vi "new control rack tester.vi"() -> ()   [LabVIEW 2011]
uses:
  <vilib>/Utility/file.llb/Write To Spreadsheet File (DBL).vi
panel:
  out "ai0 8":dynamicdata(graph) caption="Helix Limited Current Set Point"
  in  "stop":bool
  out "ai0 16":dynamicdata(graph) caption="Torroidal Current Feedback"
  out "ai0 15":dynamicdata(graph) caption="Torroidal U Limit Set Point Buffered"
  out "ai0 14":dynamicdata(graph) caption="Torroidal Voltage Feedback"
  out "ai0 13":dynamicdata(graph) caption="Torroidal Voltage Feedback"
  out "ai0 12":dynamicdata(graph) caption="ECRH Reflection"
  out "ai0 11":dynamicdata(graph) caption="ECRH Power"
  out "ai0 10":dynamicdata(graph) caption="Torroidal U Limit Set Point"
  out "ai0 9":dynamicdata(graph) caption="Torroidal Limited Current Set Point"
  out "ai0 7":dynamicdata(graph) caption="Halpha Reserve Vin/10"
  out "ai0 6":dynamicdata(graph) caption="Torroidal Limited Current Set Point"
  out "ai0 5":dynamicdata(graph) caption="Helix Limited Current Set Point"
  out "ai0 4":dynamicdata(graph) caption="Helix Voltage Feedback"
  out "ai0 3":dynamicdata(graph) caption="Helix Current Feedback"
  out "ai0 2":dynamicdata(graph) caption="Helix U Limit Set Point Buffered"
  out "ai0":dynamicdata(graph) caption="Helix U Limit Set Point"
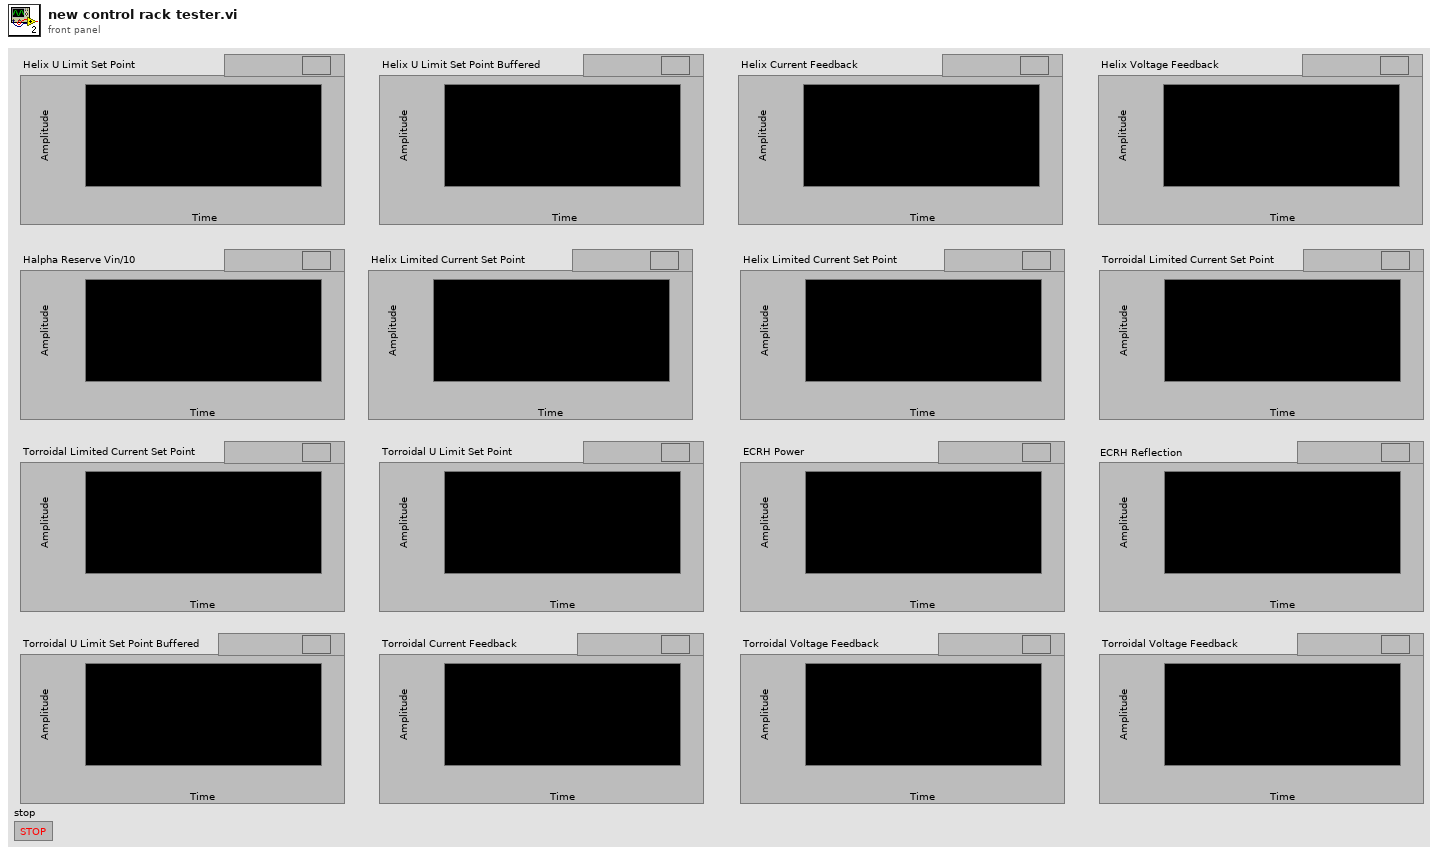
[diagram p1: front panel]
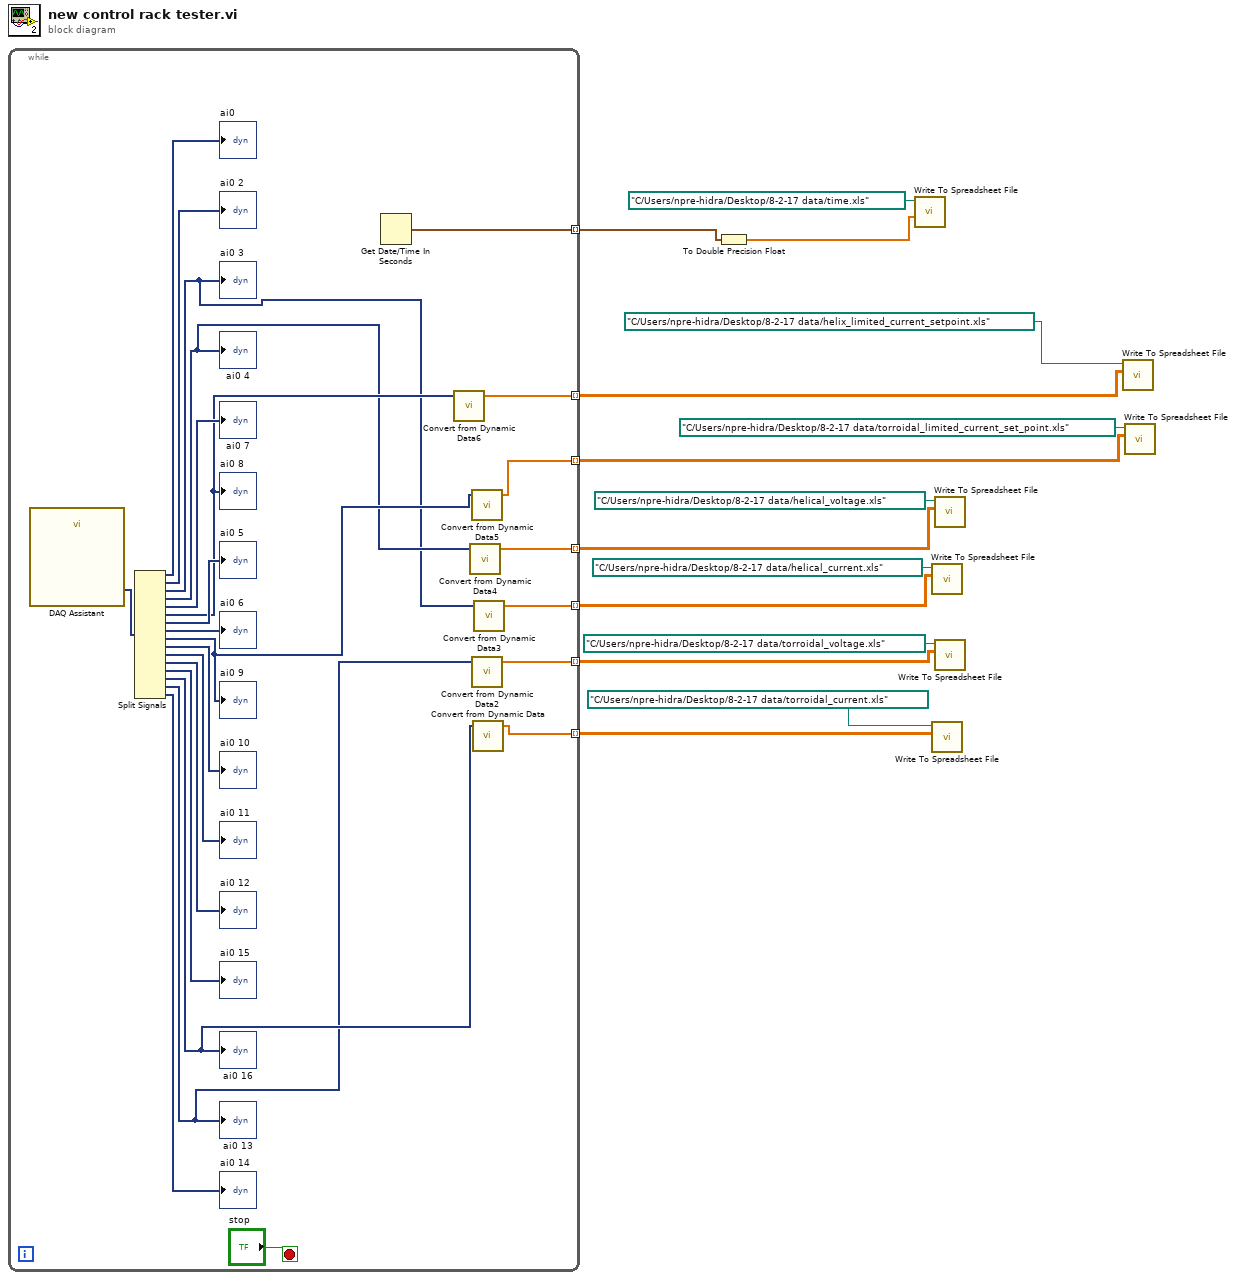
[diagram p0: block diagram]
diagram:
  n1 = while {
    tunnel: [w29] -> w14 mode=indexing
    tunnel: [w27] -> w8 mode=indexing
    tunnel: [w25] -> w6 mode=indexing
    tunnel: [w24] -> w5 mode=indexing
    tunnel: [w23] -> w4 mode=indexing
    tunnel: [w22] -> w3 mode=indexing
    tunnel: [w21] -> w2 mode=indexing
    stop <- "stop" stop-if-true
    n2 = call "DAQ Assistant"() -> ("data"=w30:dynamicdata)  [unwired: 17 in, 2 out]
    n3 = Split Signals(w30) -> (→"ai0":dynamicdata, →"ai0 2":dynamicdata, w17:dynamicdata, w18:dynamicdata, →"ai0 7":dynamicdata, w20:dynamicdata, →"ai0 5":dynamicdata, →"ai0 6":dynamicdata, w19:dynamicdata, →"ai0 10":dynamicdata, →"ai0 11":dynamicdata, →"ai0 12":dynamicdata, →"ai0 15":dynamicdata, w26:dynamicdata, w16:dynamicdata, →"ai0 14":dynamicdata)  [unwired: 16 in]
    "ai0 3" <- w17
    "ai0 4" <- w18
    "ai0 9" <- w19
    "ai0 13" <- w16
    "ai0 16" <- w26
    "ai0 8" <- w20
    n4 = Get Date/Time In Seconds() -> (seconds since 1Jan1904=w29:timestamp)
    n5 = call "Convert from Dynamic Data6"("Dynamic Data Type"=w20) -> ("Array"=w25:dbl[])  [unwired: 3 in]
    n6 = call "Convert from Dynamic Data4"("Dynamic Data Type"=w18) -> ("Array"=w23:dbl[])  [unwired: 3 in]
    n7 = call "Convert from Dynamic Data5"("Dynamic Data Type"=w19) -> ("Array"=w24:dbl[])  [unwired: 3 in]
    n8 = call "Convert from Dynamic Data2"("Dynamic Data Type"=w16) -> ("Array"=w21:dbl[])  [unwired: 3 in]
    n9 = call "Convert from Dynamic Data"("Dynamic Data Type"=w26) -> ("Array"=w27:dbl[])  [unwired: 3 in]
    n10 = call "Convert from Dynamic Data3"("Dynamic Data Type"=w17) -> ("Array"=w22:dbl[])  [unwired: 3 in]
  }
  n11 = To Double Precision Float(number=w14) -> (double precision float=w13:dbl[])
  n12 = call-poly <vilib>:"Write To Spreadsheet File.vi"("1D data"=w13, "file path (dialog if empty)"=path "C:/Users/npre-hidra/Desktop/8-2-17 data/time.xls") -> ()  [unwired: 6 in, 1 out]
  n13 = call-poly <vilib>:"Write To Spreadsheet File.vi"("2D data"=w3, "file path (dialog if empty)"=path "C:/Users/npre-hidra/Desktop/8-2-17 data/helical_current.xls") -> ()  [unwired: 6 in, 1 out]
  n14 = call-poly <vilib>:"Write To Spreadsheet File.vi"("2D data"=w8, "file path (dialog if empty)"=path "C:/Users/npre-hidra/Desktop/8-2-17 data/torroidal_current.xls") -> ()  [unwired: 6 in, 1 out]
  n15 = call-poly <vilib>:"Write To Spreadsheet File.vi"("2D data"=w4, "file path (dialog if empty)"=path "C:/Users/npre-hidra/Desktop/8-2-17 data/helical_voltage.xls") -> ()  [unwired: 6 in, 1 out]
  n16 = call-poly <vilib>:"Write To Spreadsheet File.vi"("2D data"=w2, "file path (dialog if empty)"=path "C:/Users/npre-hidra/Desktop/8-2-17 data/torroidal_voltage.xls") -> ()  [unwired: 6 in, 1 out]
  n17 = call-poly <vilib>:"Write To Spreadsheet File.vi"("2D data"=w6, "file path (dialog if empty)"=path "C:/Users/npre-hidra/Desktop/8-2-17 data/helix_limited_current_setpoint.xls") -> ()  [unwired: 6 in, 1 out]
  n18 = call-poly <vilib>:"Write To Spreadsheet File.vi"("2D data"=w5, "file path (dialog if empty)"=path "C:/Users/npre-hidra/Desktop/8-2-17 data/torroidal_limited_current_set_point.xls") -> ()  [unwired: 6 in, 1 out]
